vi "Turn on_off backlash correction.vi"(8 "error in (no error)":errorcluster, 10 "Backlash correction":bool, 11 "Lifter_motor in":refnum<class "Lifter_motor.lvclass">) -> (0 "error out":errorcluster, 3 "Lifter_motor out":refnum<class "Lifter_motor.lvclass">)   [LabVIEW 2019, in "Lifter_motor.lvclass"]
uses:
  Lifter_motor.lvclass
  Lifter_motor.lvclass/Lifter_motor.ctl
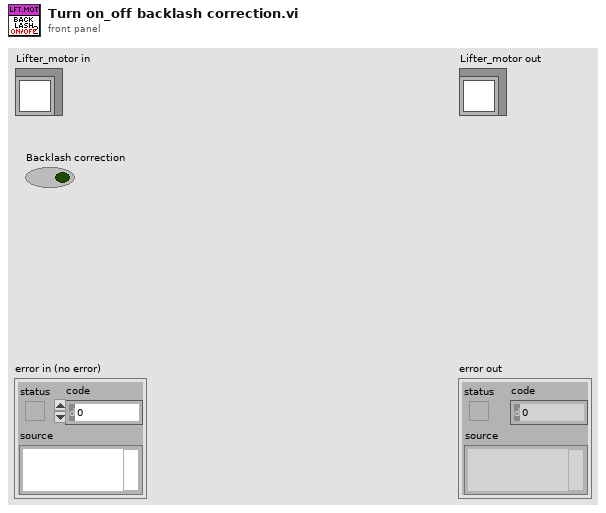
[diagram p1: front panel]
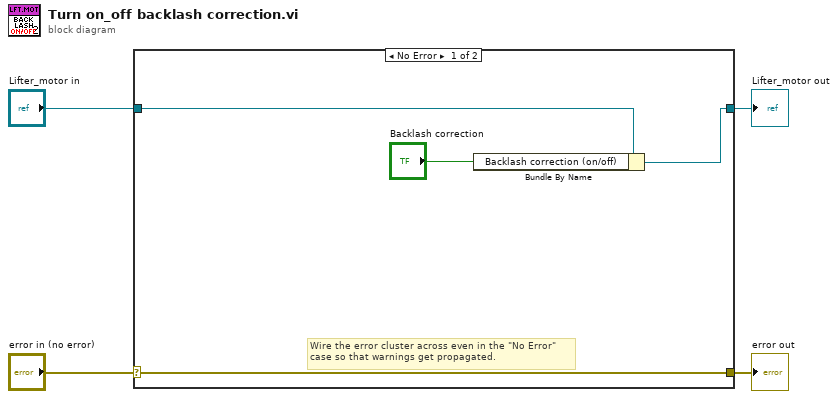
[diagram p0: block diagram]
diagram:
  n1 = case shown="No Error" "error in (no error)" {
    selector: "error in (no error)" -> [w8 w10]
    tunnel: [w8 w10] -> w3
    tunnel: [w6 w9] -> w1
    tunnel: "Lifter_motor in" -> [w7 w9]
    frame No Error {
      # "Wire the error cluster across even in the \"No Error\"\ncase so that warnings get propagated."
      n2 = Bundle By Name(cluster=w7, "Backlash correction (on/off)"="Backlash correction") -> (w6:refnum<class "Lifter_motor.lvclass">)
    }
    frame Error {
    }
  }
  "error out" <- w3
  "Lifter_motor out" <- w1
